vi "HT_RelayControl.vi"(0 "Port":string="ª\u0001&\u0000'", 1 "baud rate (9600)":u32=9600 caption="波特率(9600)", 2 "function":u16(ring) items=["OpenPort", "On", "Off", "ClosePort"], 3 "RelayIndex":u32) -> (22 "result":i32=2)   [LabVIEW 2013]
uses:
  <vilib>/Instr/_visa.llb/VISA Configure Serial Port (Instr).vi
panel:
  out "Out 2":string
  out "Out":string
  out "error out":errorcluster
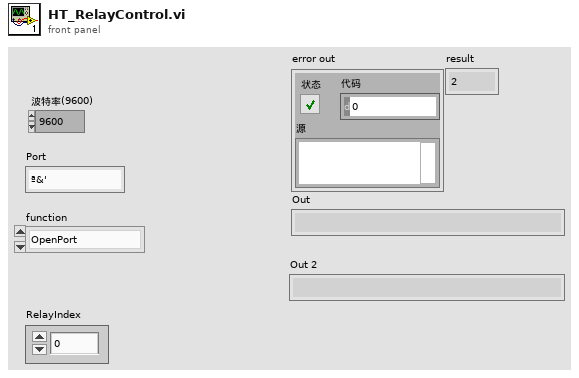
[diagram p1: front panel]
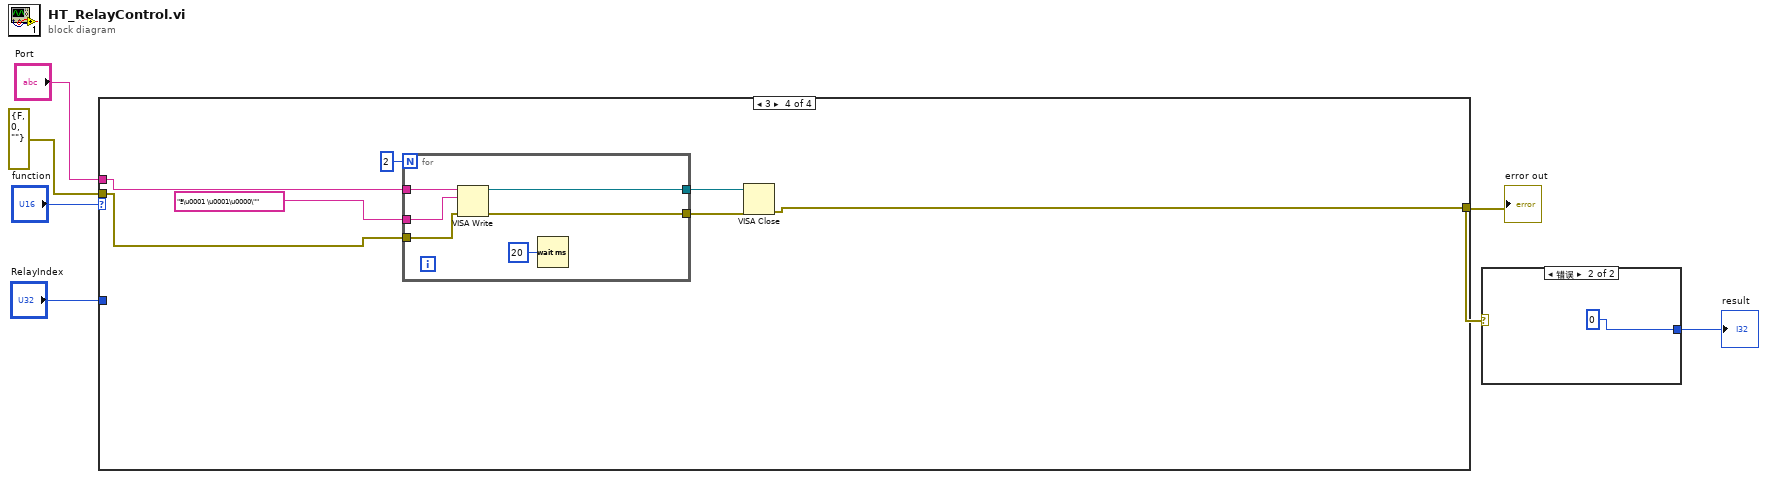
[diagram p0: block diagram]
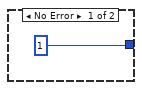
[diagram p2: hidden frame]
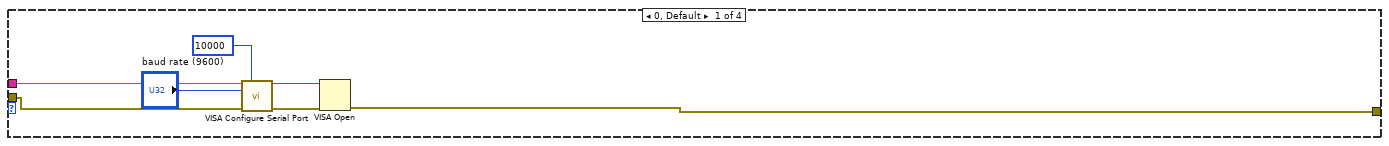
[diagram p3: hidden frame]
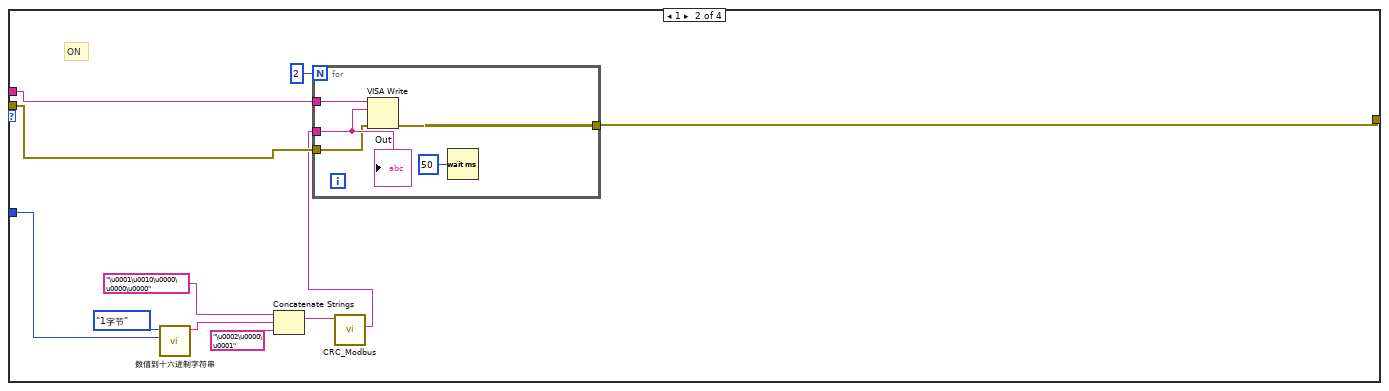
[diagram p4: hidden frame]
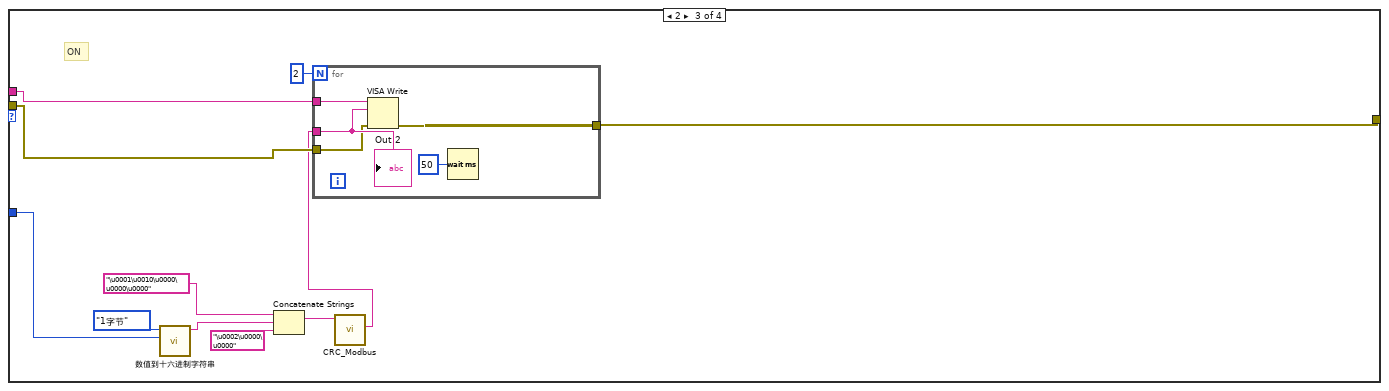
[diagram p5: hidden frame]
diagram:
  n1 = case shown="3" "function" {
    tunnel: "Port" -> [w11 w23 w39 w51]
    tunnel: errorcluster {"status"=FALSE, "code"=0, "source"=""} ("error in (no error)") -> [w10 w22 w38 w50]
    tunnel: [w9 w21 w37 w46] -> w2
    tunnel: "RelayIndex" -> [_ w19 w35 _]
    frame 0, Default {
      n2 = call-poly "VISA Configure Serial Port"("VISA resource name"=w11, "timeout (10sec)"=u32 10000, "baud rate (9600)"="baud rate (9600)", "error in (no error)"=w10) -> ("VISA resource name out"=w13:refnum<visa-resource-name>, "error out"=w12:errorcluster)  [unwired: 10 in]
      n3 = VISA Open(error in (no error)=w12, VISA resource name=w13) -> (error out=w9:errorcluster)  [unwired: 3 in, 1 out]
    }
    frame 1 {
      # "ON"
      n4 = call "数值到十六进制字符串.vi"("Numeric"=w19, "转换字节数"=enum16{"1字节", "2字节", "4字节", "3字节"}."1字节") -> ("转换结果"=w17:string)  [unwired: 8 in, 1 out]
      n5 = Concatenate Strings("\u0001\u0010\u0000\u0000\u0000" ("In"), w17, "\u0002\u0000\u0001" ("字符串")) -> (w15:string)
      n6 = call "CRC_Modbus.vi"("IN"=w15) -> ("Out"=w14:string)  [unwired: 8 in, 2 out]
      n7 = for {
        N: 2 -> [_]
        tunnel: [w29] -> w21
        tunnel: w23 -> [w28]
        tunnel: w14 -> [w27]
        tunnel: w22 -> [w26]
        n8 = VISA Write(VISA resource name=w28, write buffer=w27, error in (no error)=w26) -> (error out=w29:errorcluster)  [unwired: 2 out]
        n9 = Wait (ms)(milliseconds to wait=u32 50 ("等待时间（毫秒）")) -> ()  [unwired: 1 out]
        "Out" <- w27
      }
    }
    frame 2 {
      # "ON"
      n10 = call "数值到十六进制字符串.vi"("Numeric"=w35, "转换字节数"=enum16{"1字节", "2字节", "4字节", "3字节"}."1字节") -> ("转换结果"=w33:string)  [unwired: 8 in, 1 out]
      n11 = Concatenate Strings("\u0001\u0010\u0000\u0000\u0000" ("In"), w33, "\u0002\u0000\u0000" ("字符串")) -> (w31:string)
      n12 = call "CRC_Modbus.vi"("IN"=w31) -> ("Out"=w30:string)  [unwired: 8 in, 2 out]
      n13 = for {
        N: 2 -> [_]
        tunnel: [w45] -> w37
        tunnel: w39 -> [w44]
        tunnel: w30 -> [w43]
        tunnel: w38 -> [w42]
        n14 = VISA Write(VISA resource name=w44, write buffer=w43, error in (no error)=w42) -> (error out=w45:errorcluster)  [unwired: 2 out]
        n15 = Wait (ms)(milliseconds to wait=u32 50 ("等待时间（毫秒）")) -> ()  [unwired: 1 out]
        "Out 2" <- w43
      }
    }
    frame 3 {
      n16 = for {
        N: 2 -> [_]
        tunnel: [w58] -> w47
        tunnel: w51 -> [w57]
        tunnel: "ª\u0001 \u0001\u0000\"" ("In") -> [w56]
        tunnel: w50 -> [w55]
        tunnel: [w53] -> w48
        n17 = VISA Write(VISA resource name=w57, write buffer=w56, error in (no error)=w55) -> (VISA resource name out=w53:refnum<visa-resource-name>, error out=w58:errorcluster)  [unwired: 1 out]
        n18 = Wait (ms)(milliseconds to wait=u32 20 ("等待时间（毫秒）")) -> ()  [unwired: 1 out]
      }
      n19 = VISA Close(VISA resource name=w48, error in (no error)=w47) -> (error out=w46:errorcluster)
    }
  }
  "error out" <- w2
  n20 = case shown="错误" w2 {
    tunnel: [1 ("y") 0 ("y")] -> w1
    frame No Error {
    }
    frame Error {
    }
  }
  "result" <- w1
